vi "h.COMM.Open Connection.vi"(8 "error in":errorcluster, 9 "timeout (ms)":i32=10000, 10 "Port":T1=51971 items=["Command Socket"=51971, "Streaming Data Socket"=51972], 11 "Address":string="175.20.117.55") -> (0 "error out":errorcluster, 3 "Connection ID":refnum<k5>)   [LabVIEW 2019, in "h.Library.lvlib"]
doc: "This VI opens a socket connection to a Hyperiond Instrument\n\n<b>Address</b> - the IP address of the target Hyperion instrument\n<b>Port</b> - the socket number to open\n<b>Timeout</b> - specifies the maximum amount of time, in milliseconds, for the function to complete\n<b>error in</b> - describes error conditions that occur before this node runs. This input provides standard error functionality\n<b>Connection ID</b> - refnum of the newly established socket connection if successful\n<b>error out</b> - contains error information. This output provides standard error out functionality."
uses:
  h.Library.lvlib
  CTL/h.COMM.Socket Type.ctl
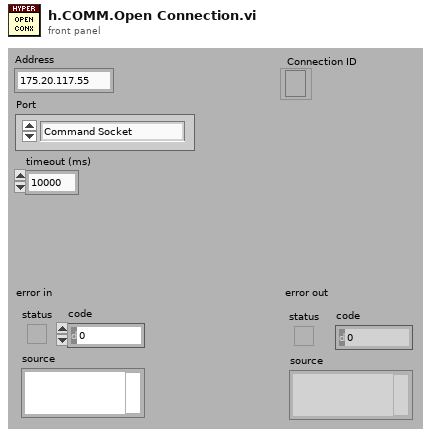
[diagram p1: front panel]
types:
  T1 = typedef "h.Library.lvlib/h.COMM.Socket Type.ctl" = u16
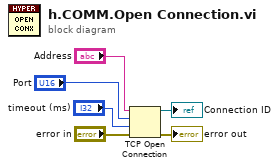
[diagram p0: block diagram]
diagram:
  n1 = TCP Open Connection(address="Address", remote port or service name="Port", timeout ms (60000)="timeout (ms)", error in (no error)="error in") -> (connection ID=→"Connection ID":refnum<k5>, error out=→"error out":errorcluster)  [unwired: 1 in]
